vi "实时小时数据单参数上传.vi"(11 "错误输入（无错误）":errorcluster) -> (4 "数据发送起始时间":timestamp format="%<%.3X\n%Y/%m/%d>T", 15 "error out":errorcluster)   [LabVIEW 2016, in "数据传输系统-03.lvlib"]
uses:
  <vilib>/Utility/config.llb/Read Key (String).vi
  <vilib>/Utility/config.llb/Write Key (String).vi
  <vilib>/Utility/config.llb/NI_LVConfig.lvlib
panel:
  out "数据拆分":bool
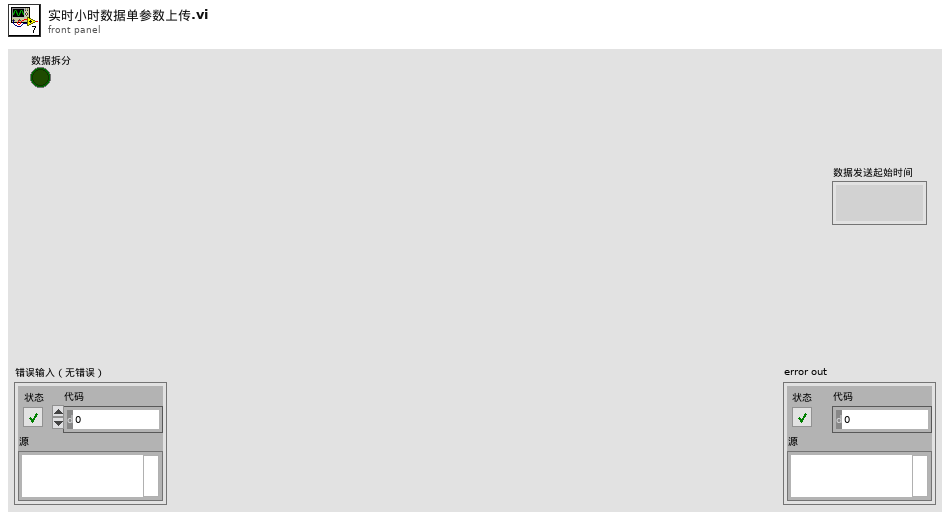
[diagram p1: front panel]
types:
  T1 = cluster{"CODMn":string, "CODCr":string, "DO":string, "铜":string, "PH":string, "氨氮":string, "比电导率":string, "水温":string, "COD":string, "浊度":string, "总氮":string, "总磷":string, "叶绿素a":string, "藻密度":string, "水位":string, "流速":string, "瞬时流量":string, "累积流量":string, "亚硝酸盐":string, "硫化物":string, "ORP":string, "铅":string, "镉":string, "锌":string, "镍":string, "锰":string, "汞":string, "气温":string, "气压":string, "风速":string, "风向":string, "盐度":string, "磷酸盐":string, "硝氮":string, "氟化物":string}
  T2 = cluster{"setini":string, "sysini":string, "hechaini":string, "actualwrite":string, "actualread":string, "datasent":string, "反控命令信息队列":string, "反控与仪器交互":string}
  T3 = typedef "NI_LVConfig.lvlib/Config Data RefNum.ctl" = refnum<k1>
  T4 = cluster{"time1":string, "time2":string, "time3":string, "time4":string, "time5":string, "time6":string, "time7":string, "time8":string, "time9":string, "time10":string, "time11":string, "time12":string, "time13":string, "time14":string, "time15":string, "time16":string, "time17":string, "time18":string, "time19":string, "time20":string, "time21":string, "time22":string, "time23":string, "time24":string, "time25":string, "time26":string, "time27":string, "time28":string, "time29":string, "time30":string, "time31":string, "time32":string, "time33":string, "time34":string, "time35":string}
  T5 = cluster{"水样数据索引[0]":string, "水样数据索引[1]":string, "水样数据索引[2]":string, "水样数据索引[3]":string, "水样数据索引[4]":string, "水样数据索引[5]":string, "水样数据索引[6]":string, "水样数据索引[7]":string, "水样数据索引[8]":string, "水样数据索引[9]":string, "水样数据索引[10]":string, "水样数据索引[11]":string, "水样数据索引[12]":string, "水样数据索引[13]":string, "水样数据索引[14]":string, "水样数据索引[15]":string, "水样数据索引[16]":string, "水样数据索引[17]":string, "水样数据索引[18]":string, "水样数据索引[19]":string, "水样数据索引[20]":string, "水样数据索引[21]":string, "水样数据索引[22]":string, "水样数据索引[23]":string, "水样数据索引[24]":string, "水样数据索引[25]":string, "水样数据索引[26]":string, "水样数据索引[27]":string, "水样数据索引[28]":string, "水样数据索引[29]":string, "水样数据索引[30]":string, "水样数据索引[31]":string, "水样数据索引[32]":string, "水样数据索引[33]":string, "水样数据索引[34]":string}
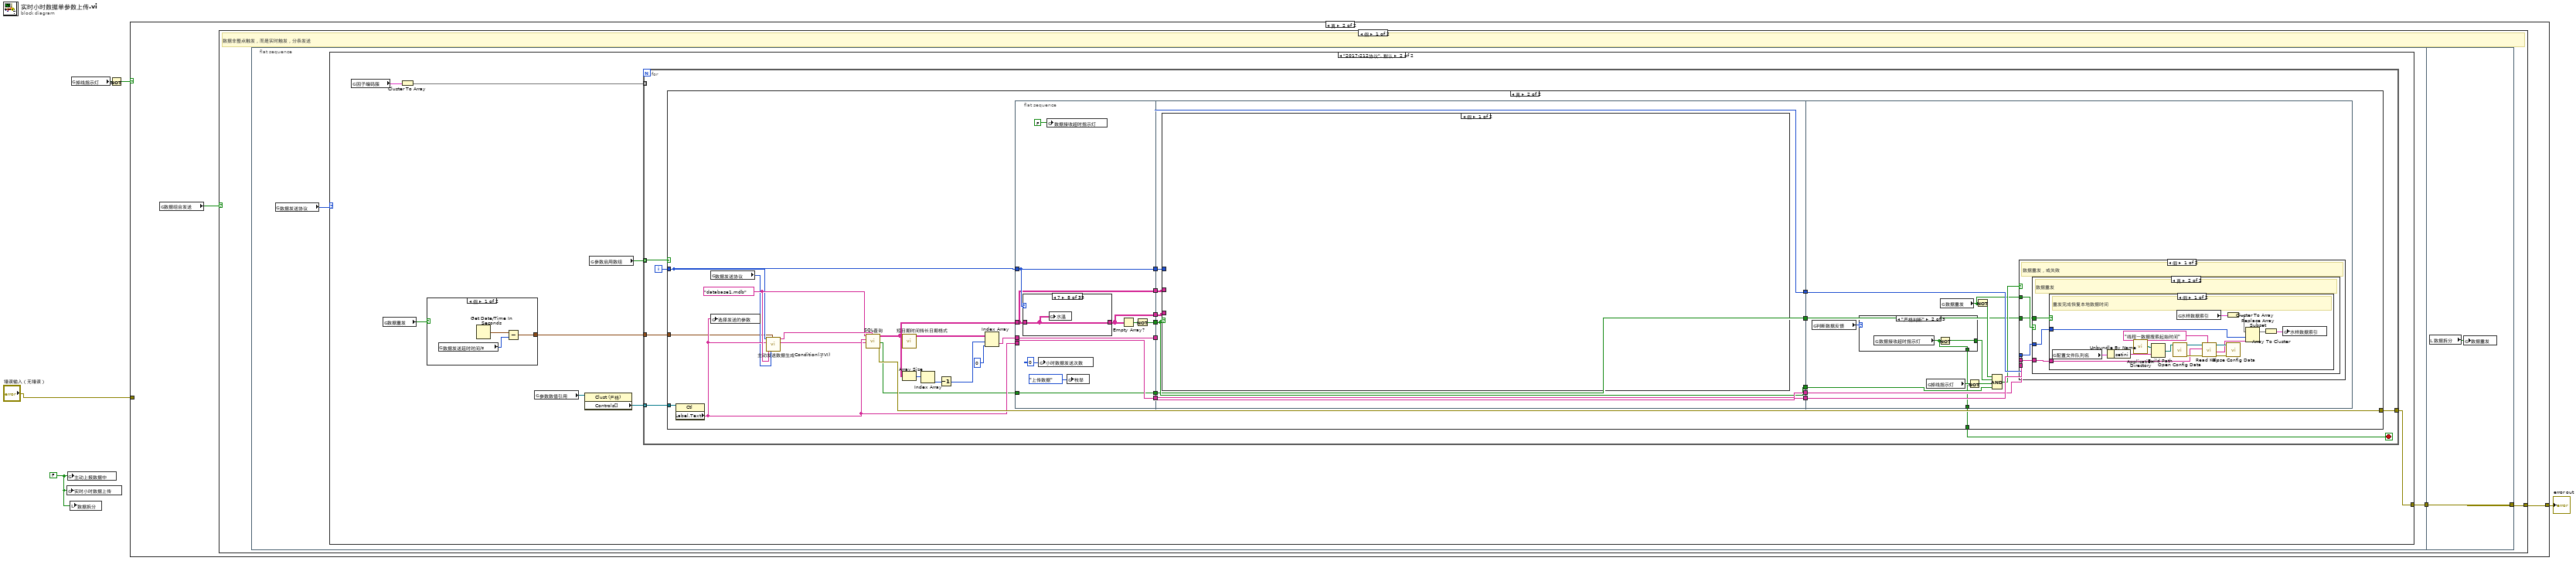
[diagram p0: block diagram]
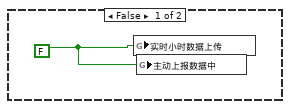
[diagram p2: hidden frame]
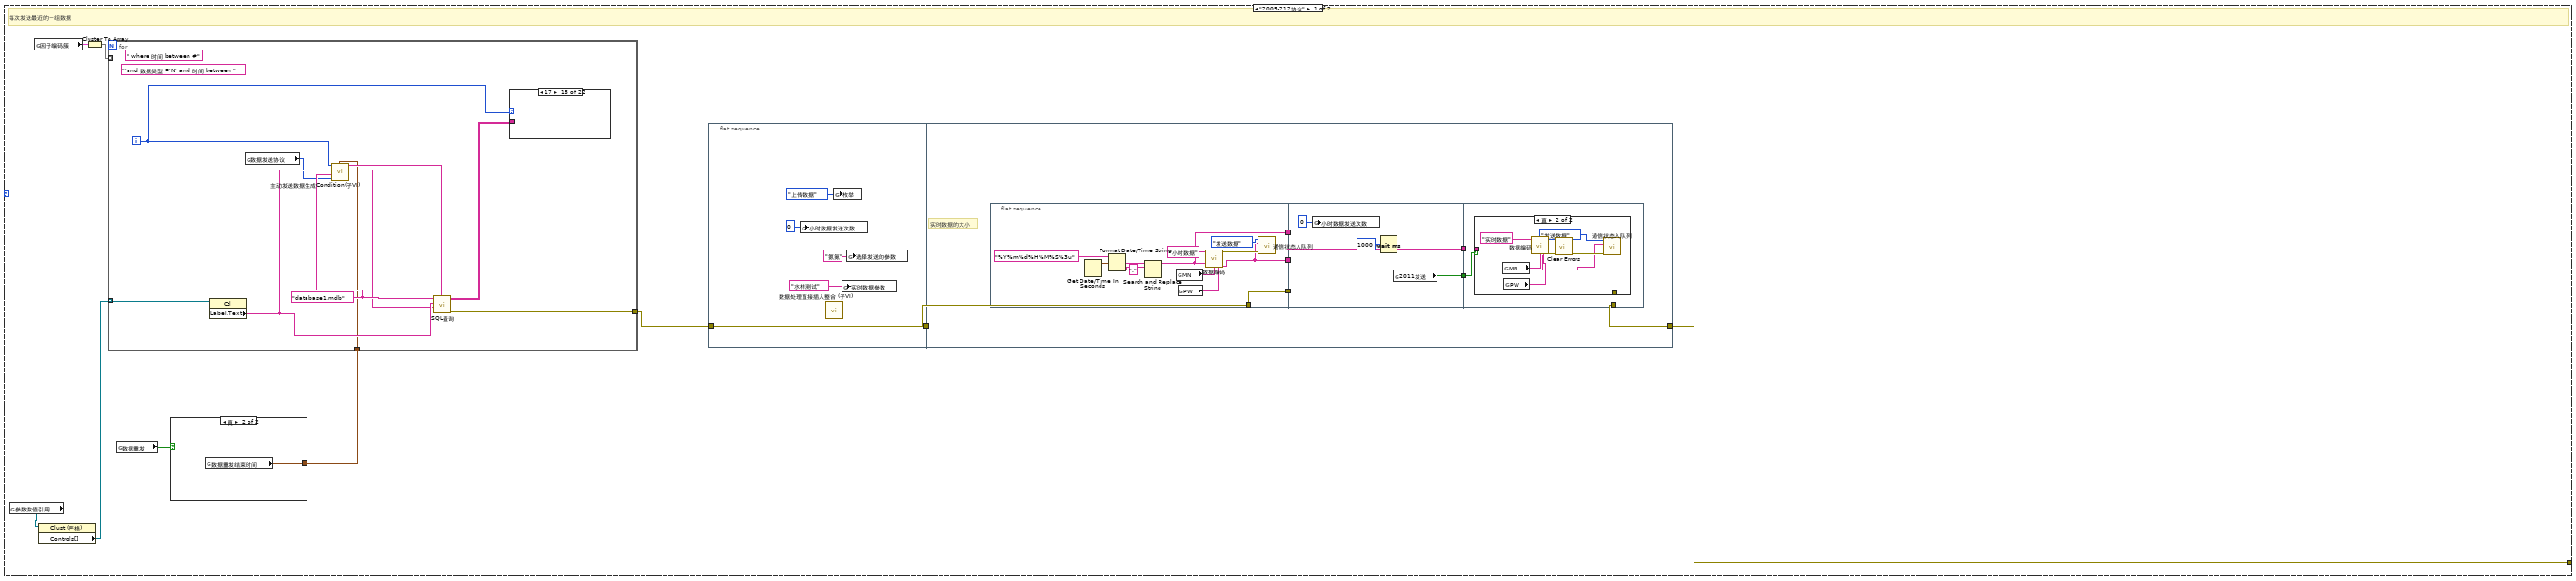
[diagram p3: hidden frame]
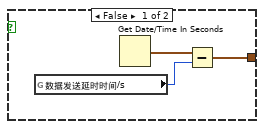
[diagram p4: hidden frame]
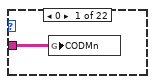
[diagram p6: hidden frame]
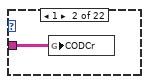
[diagram p7: hidden frame]
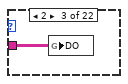
[diagram p8: hidden frame]
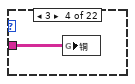
[diagram p9: hidden frame]
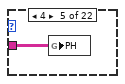
[diagram p10: hidden frame]
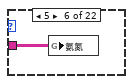
[diagram p11: hidden frame]
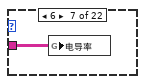
[diagram p12: hidden frame]
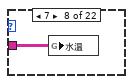
[diagram p13: hidden frame]
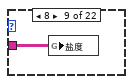
[diagram p14: hidden frame]
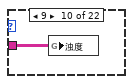
[diagram p15: hidden frame]
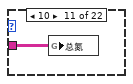
[diagram p16: hidden frame]
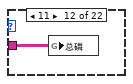
[diagram p17: hidden frame]
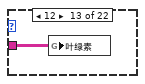
[diagram p18: hidden frame]
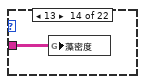
[diagram p19: hidden frame]
diagram:
  w1 = FALSE ("小时数据上传")
  n1 = global write "全局1.vi" "实时小时数据上传"(w1) -> ()
  n2 = global write "全局 数据发送重叠.vi" "主动上报数据中"(w1) -> ()
  n3 = local write "数据拆分"(w1) -> ()
  n4 = global read "全局 数据发送重叠.vi" "掉线指示灯"() -> (w5:bool)
  n5 = Not(x=w5) -> (.not. x?=w4:bool)
  n6 = case shown="真" w4 {
    tunnel: [_ w8] -> w3
    tunnel: "错误输入（无错误）" -> [_ _]
    frame False {
      w6 = FALSE ("小时数据上传")
      n7 = global write "全局1.vi" "实时小时数据上传"(w6) -> ()
      n8 = global write "全局 数据发送重叠.vi" "主动上报数据中"(w6) -> ()
    }
    frame True {
      n9 = global read "断电保存全局.vi" "数据组合发送"() -> (w7:bool)
      n10 = case shown="假" w7 {
        tunnel: [w9 _] -> w8
        frame False {
          # "数据非整点触发，而是实时触发，分条发送"
          n11 = flat-sequence {
            tunnel: [w12] -> w10
            tunnel: [w353] -> w9
            tunnel: w10 -> [w353]
            frame #0 {
              n12 = global read "断电保存全局.vi" "数据发送协议"() -> (w11:enum16{"2005-212协议", "2017-212协议"})
              n13 = case shown="\"2017-212协议\", 默认" w11 {
                tunnel: [w17 w99] -> w12
                frame "2005-212协议" {
                  # "每次发送最近的一组数据"
                  n14 = global read "断电保存全局.vi" "参数数值引用"() -> (w15:refnum<vi>)
                  n15 = global read "断电保存全局.vi" "因子编码簇"() -> (w16:T1)
                  n16 = property class="Clust (严格)"(reference=w15) -> ("Controls[]"=w18:refnum<vi>[])  [unwired: 1 in, 2 out]
                  n17 = Cluster To Array(cluster=w16) -> (array=w21:string[])
                  n18 = global read "断电保存全局.vi" "数据重发"() -> (w14:bool)
                  n19 = case shown="真" w14 {
                    tunnel: [w22 w25] -> w13
                    frame False {
                      n20 = global read "断电保存全局.vi" "数据发送延时时间/s"() -> (w23:i32)
                      n21 = Get Date/Time In Seconds() -> (seconds since 1Jan1904=w24:timestamp)
                      n22 = Subtract(x=w24, y=w23) -> (x-y=w22:timestamp)
                    }
                    frame True {
                      n23 = global read "断电保存全局.vi" "数据重发结束时间"() -> (w25:timestamp)
                    }
                  }
                  n24 = for {
                    tunnel: w21 -> [_] mode=indexing
                    tunnel: [w75] -> w20
                    tunnel: w18 -> [w70] mode=indexing
                    tunnel: w13 -> [w67]
                    i -> [w68]
                    (unwired) " where 时间 between #"
                    w73 = "database1.mdb" ("database")
                    (unwired) "'and 数据类型 ='N' and 时间 between "
                    n25 = property class="Ctl"(reference=w70) -> ("Label.Text"=w74:string)  [unwired: 1 in, 2 out]
                    n26 = global read "断电保存全局.vi" "数据发送协议"() -> (w71:enum16{"2005-212协议", "2017-212协议"})
                    n27 = call "主动发送数据生成Condition(子VI).vi"("结束时间"=w67, "数据发送协议"=w71, "database"=w73, "Label.Text"=w74, "数值"=w68) -> ("columns"=w66:string[], "CONDITION"=w72:string)  [unwired: 5 in]
                    n28 = call "SQL查询.vi"("condition"=w72, "columns"=w66, "table输入"=w74, "database"=w73) -> ("error out"=w75:errorcluster, "data"=w69:string[][])  [unwired: 4 in, 2 out]
                    n29 = case shown="17" w68 {
                      tunnel: w69 -> [w76 w77 w78 w79 w80 w81 w82 w83 w84 w85 w86 w87 w88 w89 _ _ _ _ w90 w91 w92 _]
                      frame 0 {
                        n30 = global write "全局 所有参数.vi" "CODMn"(w76) -> ()
                      }
                      frame 1 {
                        n31 = global write "全局 所有参数.vi" "CODCr"(w77) -> ()
                      }
                      frame 2 {
                        n32 = global write "全局 所有参数.vi" "DO"(w78) -> ()
                      }
                      frame 3 {
                        n33 = global write "全局 所有参数.vi" "铜"(w79) -> ()
                      }
                      frame 4 {
                        n34 = global write "全局 所有参数.vi" "PH"(w80) -> ()
                      }
                      frame 5 {
                        n35 = global write "全局 所有参数.vi" "氨氮"(w81) -> ()
                      }
                      frame 6 {
                        n36 = global write "全局 所有参数.vi" "电导率"(w82) -> ()
                      }
                      frame 7 {
                        n37 = global write "全局 所有参数.vi" "水温"(w83) -> ()
                      }
                      frame 8 {
                        n38 = global write "全局 所有参数.vi" "盐度"(w84) -> ()
                      }
                      frame 9 {
                        n39 = global write "全局 所有参数.vi" "浊度"(w85) -> ()
                      }
                      frame 10 {
                        n40 = global write "全局 所有参数.vi" "总氮"(w86) -> ()
                      }
                      frame 11 {
                        n41 = global write "全局 所有参数.vi" "总磷"(w87) -> ()
                      }
                      frame 12 {
                        n42 = global write "全局 所有参数.vi" "叶绿素"(w88) -> ()
                      }
                      frame 13 {
                        n43 = global write "全局 所有参数.vi" "藻密度"(w89) -> ()
                      }
                      frame 14 {
                      }
                      frame 15 {
                      }
                      frame 16 {
                      }
                      frame 17 {
                      }
                      frame 18 {
                        n44 = global write "全局 所有参数.vi" "亚硝酸盐"(w90) -> ()
                      }
                      frame 19 {
                        n45 = global write "全局 所有参数.vi" "硫化物"(w91) -> ()
                      }
                      frame 20 {
                        n46 = global write "全局 所有参数.vi" "ORP"(w92) -> ()
                      }
                      frame 21, Default {
                      }
                    }
                  }
                  n47 = flat-sequence {
                    tunnel: w20 -> [w26]
                    tunnel: [w26] -> w19
                    tunnel: w19 -> [w35]
                    tunnel: [w34] -> w17
                    frame #0 {
                      n48 = global write "全局 小时数据发送次数.vi" "小时数据发送次数"(0 ("小时数据发送次数")) -> ()
                      n49 = call "数据处理直接插入整合 (子VI).vi"() -> ()  [unwired: 12 in]
                      n50 = global write "全局1.vi" "枚举"(enum16{"返回请求应答", "上传数据", "返回执行结果"}."上传数据" ("枚举")) -> ()
                      n51 = global write "全局 实时数据参数.vi" "实时数据参数"("水样测试" ("实时数据参数")) -> ()
                      n52 = global write "全局 水样时间.vi" "选择发送的参数"("氨氮" ("选择发送的参数")) -> ()
                    }
                    frame #1 {
                      # "实时数据的大小"
                      n53 = flat-sequence {
                        tunnel: [w38] -> w37
                        tunnel: [w41] -> w36
                        tunnel: w35 -> [w41]
                        tunnel: [w40] -> w33
                        tunnel: w37 -> [_]
                        tunnel: w36 -> [_]
                        tunnel: w33 -> [w51]
                        tunnel: [w51] -> w32
                        tunnel: [w50] -> w31
                        tunnel: [w56] -> w34
                        tunnel: w32 -> [w55]
                        tunnel: w31 -> [w54]
                        frame #0 {
                          n54 = Get Date/Time In Seconds() -> (seconds since 1Jan1904=w47:timestamp)
                          n55 = Format Date/Time String(time format string (%c)="%Y%m%d%H%M%S%3u" ("时间格式字符串(%c)"), seconds (now)=w47) -> (date/time string=w48:string)  [unwired: 1 in]
                          n56 = Search and Replace String(input string=w48, search string="." ("搜索字符串")) -> (result string=w40:string)  [unwired: 6 in, 3 out]
                          n57 = global read "断电保存全局.vi" "MN"() -> (w44:string)
                          n58 = global read "断电保存全局.vi" "PW"() -> (w43:string)
                          n59 = call "数据编码.vi"("table输入"="小时数据" ("新元素/子数组"), "QN"=w40, "MN"=w44, "PW"=w43) -> ("错误常量"=w42:errorcluster, "通讯包字符串"=w38:string)  [unwired: 10 in]
                          n60 = call "通信状态入队列.vi"("错误输入（无错误）"=w42, "发送报文"=w38, "枚举"=enum16{"打开连接", "发送数据", "读取数据", "数据处理", "关闭连接"}."发送数据") -> ()  [unwired: 8 in, 1 out]
                        }
                        frame #1 {
                          n61 = global write "全局 小时数据发送次数.vi" "小时数据发送次数"(0 ("小时数据发送次数")) -> ()
                          n62 = Wait (ms)(milliseconds to wait=u32 1000 ("等待时间（毫秒）")) -> ()  [unwired: 1 out]
                          n63 = global read "断电保存全局.vi" "2011发送"() -> (w50:bool)
                        }
                        frame #2 {
                          n64 = case shown="真" w54 {
                            tunnel: [_ w61] -> w56
                            tunnel: w55 -> [_ w60]
                            frame False {
                            }
                            frame True {
                              n65 = global read "断电保存全局.vi" "MN"() -> (w63:string)
                              n66 = global read "断电保存全局.vi" "PW"() -> (w64:string)
                              n67 = call "数据编码.vi"("table输入"="实时数据" ("新元素/子数组"), "QN"=w60, "MN"=w63, "PW"=w64) -> ("错误常量"=w62:errorcluster, "通讯包字符串"=w57:string)  [unwired: 10 in]
                              n68 = call <vilib>:"Clear Errors.vi"("error in (no error)"=w62) -> ("error out"=w59:errorcluster)  [unwired: 5 in, 1 out]
                              n69 = call "通信状态入队列.vi"("错误输入（无错误）"=w59, "发送报文"=w57, "枚举"=enum16{"打开连接", "发送数据", "读取数据", "数据处理", "关闭连接"}."发送数据") -> ("错误输出"=w61:errorcluster)  [unwired: 8 in]
                            }
                          }
                        }
                      }
                    }
                  }
                }
                frame "2017-212协议", Default {
                  n70 = global read "断电保存全局.vi" "因子编码簇"() -> (w97:T1)
                  n71 = global read "断电保存全局.vi" "数据重发"() -> (w94:bool)
                  n72 = Cluster To Array(cluster=w97) -> (array=w100:string[])
                  n73 = case shown="假" w94 {
                    tunnel: [w101 w104] -> w93
                    frame False {
                      n74 = global read "断电保存全局.vi" "数据发送延时时间/s"() -> (w102:i32)
                      n75 = Get Date/Time In Seconds() -> (seconds since 1Jan1904=w103:timestamp)
                      n76 = Subtract(x=w103, y=w102) -> (x-y=w101:timestamp)
                    }
                    frame True {
                      n77 = global read "断电保存全局.vi" "数据重发结束时间"() -> (w104:timestamp)
                    }
                  }
                  n78 = global read "断电保存全局.vi" "参数数值引用"() -> (w96:refnum<vi>)
                  n79 = property class="Clust (严格)"(reference=w96) -> ("Controls[]"=w98:refnum<vi>[])  [unwired: 1 in, 2 out]
                  n80 = global read "断电保存全局.vi" "参数启用数组"() -> (w95:bool[])
                  n81 = for {
                    tunnel: w100 -> [_] mode=indexing
                    tunnel: [w110] -> w99
                    tunnel: w98 -> [w108] mode=indexing
                    tunnel: w95 -> [w107] mode=indexing
                    tunnel: w93 -> [w106]
                    i -> [w109]
                    stop <- w105 stop-if-true
                    n82 = case shown="真" w107 {
                      tunnel: [_ w129] -> w110
                      tunnel: w109 -> [_ w120]
                      tunnel: w108 -> [_ w119]
                      tunnel: w106 -> [_ w116]
                      tunnel: [_ w114] -> w105
                      frame False {
                      }
                      frame True {
                        w128 = "database1.mdb" ("database")
                        n83 = property class="Ctl"(reference=w119) -> ("Label.Text"=w127:string)  [unwired: 1 in, 2 out]
                        n84 = global read "断电保存全局.vi" "数据发送协议"() -> (w126:enum16{"2005-212协议", "2017-212协议"})
                        n85 = global write "全局 水样时间.vi" "选择发送的参数"(w127) -> ()
                        n86 = call "主动发送数据生成Condition(子VI).vi"("结束时间"=w116, "数据发送协议"=w126, "database"=w128, "Label.Text"=w127, "数值"=w120) -> ("columns"=w118:string[], "CONDITION"=w132:string)  [unwired: 5 in]
                        n87 = call "SQL查询.vi"("condition"=w132, "columns"=w118, "table输入"=w127, "database"=w128) -> ("error out"=w129:errorcluster, "拆分数据"=w112:bool, "data"=w123:string[][])  [unwired: 4 in, 1 out]
                        n88 = call "短日期时间转长日期格式.vi"("data"=w123) -> ("输出数组"=w131:string[][])  [unwired: 10 in]
                        n89 = Array Size(array=w123) -> (size(s)=w125:i32[])
                        n90 = Index Array(array=w125) -> (element=w124:i32)  [unwired: 1 in]
                        n91 = Decrement(x=w124) -> (x-1=w122:i32)
                        n92 = Index Array(array=w131, index (row)=w122, index (col)=0 ("禁用的索引 (列)")) -> (element=w130:string)
                        n93 = flat-sequence {
                          tunnel: [w144] -> w140
                          tunnel: [w143] -> w139
                          tunnel: w123 -> [w142]
                          tunnel: w120 -> [w147]
                          tunnel: w127 -> [w149]
                          tunnel: [w149] -> w138
                          tunnel: w130 -> [w148]
                          tunnel: [w148] -> w137
                          tunnel: [w147] -> w136
                          tunnel: [w142] -> w115
                          tunnel: [w141] -> w113
                          tunnel: w112 -> [w141]
                          tunnel: w140 -> [w189]
                          tunnel: w139 -> [w193]
                          tunnel: [w192] -> w135
                          tunnel: w138 -> [w192]
                          tunnel: [w191] -> w134
                          tunnel: w137 -> [w191]
                          tunnel: [w190] -> w133
                          tunnel: w136 -> [w190]
                          tunnel: [w189] -> w117
                          tunnel: w115 -> [w188]
                          tunnel: w113 -> [w187]
                          tunnel: [w187] -> w111
                          tunnel: w135 -> [w302]
                          tunnel: w134 -> [w301]
                          tunnel: w133 -> [w300]
                          tunnel: w117 -> [w299]
                          tunnel: [w291] -> w114
                          tunnel: w111 -> [w290]
                          frame #0 {
                            n94 = case shown="7" w147 {
                              tunnel: w142 -> [w152 w153 w154 w155 w156 w157 w158 w159 w160 w161 w162 w163 w164 w165 _ _ _ _ w170 w171 w172 w173 w174 w175 w176 w177 w178 _ _ _ _ w183 w184 w185 w186]
                              tunnel: [w152 w153 w154 w155 w156 w157 w158 w159 w160 w161 w162 w163 w164 w165 w166 w167 w168 w169 w170 w171 w172 w173 w174 w175 w176 w177 w178 w179 w180 w181 w182 w183 w184 w185 w186] -> w143
                              frame 0, Default {
                                n95 = global write "全局 所有参数.vi" "CODMn"(w152) -> ()
                              }
                              frame 1 {
                                n96 = global write "全局 所有参数.vi" "CODCr"(w153) -> ()
                              }
                              frame 2 {
                                n97 = global write "全局 所有参数.vi" "DO"(w154) -> ()
                              }
                              frame 3 {
                                n98 = global write "全局 所有参数.vi" "铜"(w155) -> ()
                              }
                              frame 4 {
                                n99 = global write "全局 所有参数.vi" "PH"(w156) -> ()
                              }
                              frame 5 {
                                n100 = global write "全局 所有参数.vi" "氨氮"(w157) -> ()
                              }
                              frame 6 {
                                n101 = global write "全局 所有参数.vi" "电导率"(w158) -> ()
                              }
                              frame 7 {
                                n102 = global write "全局 所有参数.vi" "水温"(w159) -> ()
                              }
                              frame 8 {
                                n103 = global write "全局 所有参数.vi" "盐度"(w160) -> ()
                              }
                              frame 9 {
                                n104 = global write "全局 所有参数.vi" "浊度"(w161) -> ()
                              }
                              frame 10 {
                                n105 = global write "全局 所有参数.vi" "总氮"(w162) -> ()
                              }
                              frame 11 {
                                n106 = global write "全局 所有参数.vi" "总磷"(w163) -> ()
                              }
                              frame 12 {
                                n107 = global write "全局 所有参数.vi" "叶绿素"(w164) -> ()
                              }
                              frame 13 {
                                n108 = global write "全局 所有参数.vi" "藻密度"(w165) -> ()
                              }
                              frame 14 {
                                n109 = global read "全局 所有参数.vi" "水位"() -> (w166:string[][])
                              }
                              frame 15 {
                                n110 = global read "全局 所有参数.vi" "流速"() -> (w167:string[][])
                              }
                              frame 16 {
                                n111 = global read "全局 所有参数.vi" "瞬时流量"() -> (w168:string[][])
                              }
                              frame 17 {
                                n112 = global read "全局 所有参数.vi" "累积流量"() -> (w169:string[][])
                              }
                              frame 18 {
                                n113 = global write "全局 所有参数.vi" "亚硝酸盐"(w170) -> ()
                              }
                              frame 19 {
                                n114 = global write "全局 所有参数.vi" "硫化物"(w171) -> ()
                              }
                              frame 20 {
                                n115 = global write "全局 所有参数.vi" "ORP"(w172) -> ()
                              }
                              frame 21 {
                                n116 = global write "全局 所有参数.vi" "铅"(w173) -> ()
                              }
                              frame 22 {
                                n117 = global write "全局 所有参数.vi" "镉"(w174) -> ()
                              }
                              frame 23 {
                                n118 = global write "全局 所有参数.vi" "锌"(w175) -> ()
                              }
                              frame 24 {
                                n119 = global write "全局 所有参数.vi" "镍"(w176) -> ()
                              }
                              frame 25 {
                                n120 = global write "全局 所有参数.vi" "锰"(w177) -> ()
                              }
                              frame 26 {
                                n121 = global write "全局 所有参数.vi" "汞"(w178) -> ()
                              }
                              frame 27 {
                                n122 = global read "全局 所有参数.vi" "气温"() -> (w179:string[][])
                              }
                              frame 28 {
                                n123 = global read "全局 所有参数.vi" "气压"() -> (w180:string[][])
                              }
                              frame 29 {
                                n124 = global read "全局 所有参数.vi" "风速"() -> (w181:string[][])
                              }
                              frame 30 {
                                n125 = global read "全局 所有参数.vi" "风向"() -> (w182:string[][])
                              }
                              frame 31 {
                                n126 = global write "全局 所有参数.vi" "盐度 2"(w183) -> ()
                              }
                              frame 32 {
                                n127 = global write "全局 所有参数.vi" "磷酸盐"(w184) -> ()
                              }
                              frame 33 {
                                n128 = global write "全局 所有参数.vi" "硝氮"(w185) -> ()
                              }
                              frame 34 {
                                n129 = global write "全局 所有参数.vi" "氟化物"(w186) -> ()
                              }
                            }
                            n130 = global write "全局 小时数据发送次数.vi" "小时数据发送次数"(0 ("小时数据发送次数")) -> ()
                            n131 = global write "全局 数据发送重叠.vi" "数据接收超时指示灯"(FALSE ("数据接收超时指示灯")) -> ()
                            n132 = global write "全局1.vi" "枚举"(enum16{"返回请求应答", "上传数据", "返回执行结果"}."上传数据" ("枚举")) -> ()
                            n133 = Empty Array?(array=w143) -> (empty?=w145:bool)
                            n134 = Not(x=w145) -> (.not. x?=w144:bool)
                          }
                          frame #1 {
                            n135 = case shown="假" w189 {
                              tunnel: w193 -> [_ w198]
                              tunnel: w190 -> [_ w197]
                              tunnel: w188 -> [_ w195]
                              frame False {
                              }
                              frame True {
                                n136 = flat-sequence {
                                tunnel: w198 -> [w201]
                                tunnel: [w201] -> w196
                                tunnel: w195 -> [w199]
                                tunnel: [w199] -> w194
                                tunnel: w197 -> [w203]
                                tunnel: w196 -> [w204]
                                tunnel: w194 -> [w202]
                                frame #0 {
                                w200 = TRUE ("小时数据上传")
                                n137 = global write "全局 数据发送重叠.vi" "主动上报数据中"(w200) -> ()
                                n138 = global write "全局1.vi" "实时小时数据上传"(w200) -> ()
                                }
                                frame #1 {
                                n139 = case shown="0, 默认" w203 {
                                selector: w203 -> [w205 _]
                                tunnel: w203 -> [_ w236]
                                tunnel: w204 -> [w208 w235]
                                tunnel: w202 -> [w207 w234]
                                frame 14..17, 27..30 {
                                n140 = for {
                                tunnel: [w232] -> w209
                                tunnel: w205 -> [w231]
                                tunnel: w208 -> [_] mode=indexing
                                i -> [w233]
                                stop <- w230 stop-if-true
                                n141 = call "小时数据发送 (子VI).vi"("数值"=w231) -> ("error out"=w232:errorcluster, "超时退出"=w230:bool)  [unwired: 9 in]
                                n142 = global write "全局 小时数据发送次数.vi" "小时数据发送次数"(w233) -> ()
                                }
                                n143 = global read "断电保存全局.vi" "2011发送"() -> (w206:bool)
                                n144 = case shown="真" w206 {
                                tunnel: w209 -> [_ w214]
                                tunnel: w205 -> [_ w213]
                                tunnel: w207 -> [_ w212]
                                tunnel: w205 -> [_ w210]
                                frame False {
                                }
                                frame True {
                                n145 = flat-sequence {
                                tunnel: w214 -> [w218]
                                tunnel: [w218] -> w215
                                tunnel: w213 -> [w217]
                                tunnel: w212 -> [w216]
                                tunnel: [w216] -> w211
                                frame #0 {
                                n146 = case shown="27" w217 {
                                tunnel: w216 -> [_ w219 w220 w221 w222 w223 w224 w225 w226]
                                frame 0, Default {
                                }
                                frame 14 {
                                n147 = global write "全局 所有参数.vi" "水位"(w219) -> ()
                                }
                                frame 15 {
                                n148 = global write "全局 所有参数.vi" "流速"(w220) -> ()
                                }
                                frame 16 {
                                n149 = global write "全局 所有参数.vi" "瞬时流量"(w221) -> ()
                                }
                                frame 17 {
                                n150 = global write "全局 所有参数.vi" "累积流量"(w222) -> ()
                                }
                                frame 27 {
                                n151 = global write "全局 所有参数.vi" "气温"(w223) -> ()
                                }
                                frame 28 {
                                n152 = global write "全局 所有参数.vi" "气压"(w224) -> ()
                                }
                                frame 29 {
                                n153 = global write "全局 所有参数.vi" "风速"(w225) -> ()
                                }
                                frame 30 {
                                n154 = global write "全局 所有参数.vi" "风向"(w226) -> ()
                                }
                                }
                                }
                                }
                                n155 = for {
                                tunnel: w215 -> [_]
                                tunnel: w211 -> [_] mode=indexing
                                tunnel: w210 -> [w228]
                                i -> [w229]
                                stop <- w227 stop-if-true
                                n156 = global write "全局 小时数据发送次数.vi" "小时数据发送次数"(w229) -> ()
                                n157 = call "实时数据发送 (子VI).vi"("数值"=w228) -> ("超时退出"=w227:bool)  [unwired: 10 in]
                                }
                                }
                                }
                                }
                                frame 0, Default {
                                n158 = for {
                                tunnel: w236 -> [w239]
                                tunnel: w235 -> [w245] mode=indexing
                                tunnel: w234 -> [w241]
                                i -> [w240]
                                stop <- w237 stop-if-true
                                n159 = Index Array(array=w245, index #1=1 ("索引"), index #2=2 ("索引")) -> (element #1=w238:string, element #2=w242:string)
                                n160 = global write "全局 小时数据发送次数.vi" "小时数据发送次数"(w240) -> ()
                                n161 = case shown="\"水样测试\"" w238 {
                                tunnel: w239 -> [_ w249 _ _ _]
                                tunnel: w242 -> [_ w248 w281 w284 w287]
                                tunnel: w241 -> [_ w247 _ _ _]
                                tunnel: [_ w246 w280 w283 w286] -> w237
                                frame "假", Default {
                                }
                                frame "水样测试" {
                                n162 = case shown="\"hd\", \"N\", 默认" w248 {
                                tunnel: w249 -> [w253 w274]
                                tunnel: w247 -> [w252 w273]
                                tunnel: [w250 w271] -> w246
                                frame "M" {
                                n163 = global read "断电保存全局.vi" "2011发送"() -> (w251:bool)
                                n164 = case shown="真" w251 {
                                tunnel: w253 -> [_ w256]
                                tunnel: w252 -> [_ w255]
                                tunnel: [_ w254] -> w250
                                frame False {
                                }
                                frame True {
                                n165 = flat-sequence {
                                tunnel: w256 -> [w258]
                                tunnel: w255 -> [w259]
                                tunnel: [w258] -> w257
                                tunnel: w257 -> [w269]
                                tunnel: [w268] -> w254
                                frame #0 {
                                n166 = case shown="14" w258 {
                                tunnel: w259 -> [_ w260 w261 w262 w263 w264 w265 w266 w267]
                                frame 0, Default {
                                }
                                frame 14 {
                                n167 = global write "全局 所有参数.vi" "水位"(w260) -> ()
                                }
                                frame 15 {
                                n168 = global write "全局 所有参数.vi" "流速"(w261) -> ()
                                }
                                frame 16 {
                                n169 = global write "全局 所有参数.vi" "瞬时流量"(w262) -> ()
                                }
                                frame 17 {
                                n170 = global write "全局 所有参数.vi" "累积流量"(w263) -> ()
                                }
                                frame 27 {
                                n171 = global write "全局 所有参数.vi" "气温"(w264) -> ()
                                }
                                frame 28 {
                                n172 = global write "全局 所有参数.vi" "气压"(w265) -> ()
                                }
                                frame 29 {
                                n173 = global write "全局 所有参数.vi" "风速"(w266) -> ()
                                }
                                frame 30 {
                                n174 = global write "全局 所有参数.vi" "风向"(w267) -> ()
                                }
                                }
                                }
                                frame #1 {
                                n175 = call "实时数据发送 (子VI).vi"("数值"=w269) -> ("超时退出"=w268:bool)  [unwired: 10 in]
                                }
                                }
                                }
                                }
                                }
                                frame "hd", "N", Default {
                                n176 = call "小时数据发送 (子VI).vi"("数值"=w274) -> ("error out"=w272:errorcluster, "超时退出"=w270:bool)  [unwired: 9 in]
                                n177 = global read "断电保存全局.vi" "2011发送"() -> (w275:bool)
                                n178 = case shown="真" w275 {
                                tunnel: w274 -> [_ w279]
                                tunnel: w273 -> [_ _]
                                tunnel: w272 -> [_ _]
                                tunnel: [_ w276] -> w271
                                tunnel: w270 -> [_ w278]
                                frame False {
                                }
                                frame True {
                                n179 = call "实时数据发送 (子VI).vi"("数值"=w279) -> ("超时退出"=w277:bool)  [unwired: 10 in]
                                n180 = Or(x=w278, y=w277) -> (x .or. y?=w276:bool)
                                }
                                }
                                }
                                }
                                }
                                frame "空白测试", "零点核查" {
                                n181 = case shown="\"N\", 默认" w281 {
                                tunnel: [_ w282] -> w280
                                frame "M" {
                                }
                                frame "N", Default {
                                n182 = call "零点核查数据发送 (子VI).vi"() -> ("超时退出"=w282:bool)  [unwired: 11 in]
                                }
                                }
                                }
                                frame "跨度核查" {
                                n183 = case shown="\"N\", 默认" w284 {
                                tunnel: [_ w285] -> w283
                                frame "M" {
                                }
                                frame "N", Default {
                                n184 = call "跨度核查数据发送 (子VI).vi"() -> ("超时退出"=w285:bool)  [unwired: 11 in]
                                }
                                }
                                }
                                frame "标样核查" {
                                n185 = case shown="\"N\", 默认" w287 {
                                tunnel: [_ w288] -> w286
                                frame "M" {
                                }
                                frame "N", Default {
                                n186 = call "标样核查数据发送(子VI).vi"() -> ("超时退出"=w288:bool)  [unwired: 11 in]
                                }
                                }
                                }
                                }
                                }
                                }
                                }
                                }
                                frame #2 {
                                w289 = FALSE ("小时数据上传")
                                n187 = global write "全局 数据发送重叠.vi" "主动上报数据中"(w289) -> ()
                                n188 = global write "全局1.vi" "实时小时数据上传"(w289) -> ()
                                }
                                }
                              }
                            }
                          }
                          frame #2 {
                            n189 = global read "断电保存全局.vi" "判断数据反馈"() -> (w296:enum16{"非严格判断", "严格判断", "不判断"})
                            n190 = case shown="\"严格判断\"" w296 {
                              tunnel: [TRUE w306 TRUE] -> w295
                              tunnel: [FALSE ("数据接收超时指示灯") w305 FALSE ("数据接收超时指示灯")] -> w291
                              frame "非严格判断", Default {
                              }
                              frame "严格判断" {
                                n191 = global read "全局 数据发送重叠.vi" "数据接收超时指示灯"() -> (w305:bool)
                                n192 = Not(x=w305) -> (.not. x?=w306:bool)
                              }
                              frame "不判断" {
                              }
                            }
                            n193 = global read "全局 数据发送重叠.vi" "掉线指示灯"() -> (w298:bool)
                            n194 = global read "断电保存全局.vi" "数据重发"() -> (w292:bool)
                            n195 = Not(x=w298) -> (.not. x?=w297:bool)
                            n196 = Not(x=w292) -> (.not. x?=w293:bool)
                            n197 = Compound Arithmetic op=AND ("复合运算")(w293, w295, w297, w299) -> (w294:bool)
                            n198 = case shown="假" w294 {
                              tunnel: w301 -> [_ w343]
                              tunnel: w300 -> [w310 w337]
                              tunnel: w302 -> [w312 w344]
                              tunnel: w292 -> [w311 _]
                              tunnel: w290 -> [w309 _]
                              frame False {
                                # "数据重发，或失败"
                                n199 = case shown="真" w311 {
                                tunnel: w312 -> [_ w315]
                                tunnel: w310 -> [_ w314]
                                tunnel: w309 -> [_ w313]
                                frame False {
                                # "数据发送失败"
                                }
                                frame True {
                                # "数据重发"
                                n200 = case shown="假" w313 {
                                tunnel: w315 -> [w318 _]
                                tunnel: w314 -> [w316 _]
                                frame False {
                                # "重发完成恢复本地数据时间"
                                n201 = global read "断电保存全局.vi" "配置文件队列名"() -> (w325:T2)
                                n202 = Unbundle By Name(w325) -> ("setini"=w326:string)
                                n203 = call <vilib>:"Application Directory.vi"() -> ("Application Directory"=w319:path)
                                n204 = Build Path(base path=w319, name or relative path=w326) -> (appended path=w320:path)
                                n205 = call <vilib>:"Open Config Data.vi"("configuration file path"=w320) -> ("error out"=w327:errorcluster, "refnum"=w321:T3)  [unwired: 8 in, 1 out]
                                n206 = global read "全局 水样时间.vi" "水样数据索引"() -> (w328:T4)
                                n207 = call-poly <vilib>:"Read Key.vi"("section"="线程一数据搜索起始时间", "error in (no error)"=w327, "key"=w318, "refnum"=w321) -> ("error out"=w324:errorcluster, "value"=w317:string, "refnum out"=w323:T3)  [unwired: 4 in, 1 out]
                                n208 = Cluster To Array(cluster=w328) -> (array=w329:string[])
                                n209 = call <vilib>:"Close Config Data.vi"("error in (no error)"=w324, "refnum"=w323) -> ()  [unwired: 8 in, 2 out]
                                n210 = Replace Array Subset(array=w329, new element=w317, index=w316) -> (w330:string[])
                                n211 = Array To Cluster(array=w330) -> (cluster=w331:T5)
                                n212 = global write "全局 水样时间.vi" "水样数据索引"(w331) -> ()
                                }
                                frame True {
                                # "数据拆分，继续重发"
                                "数据拆分" <- TRUE
                                }
                                }
                                }
                                }
                              }
                              frame True {
                                # "保存本地"
                                n213 = global read "断电保存全局.vi" "配置文件队列名"() -> (w334:T2)
                                n214 = call "日期时间字符串转换分钟数加一.vi"("枚举"=enum16{"分钟数加一", "秒数加一", "小时数加一"}."秒数加一", "data[0]"=w343) -> ("日期/时间字符串"=w336:string)  [unwired: 9 in]
                                n215 = Unbundle By Name(w334) -> ("setini"=w333:string)
                                n216 = global read "全局 水样时间.vi" "水样数据索引"() -> (w338:T4)
                                n217 = call <vilib>:"Application Directory.vi"() -> ("Application Directory"=w345:path)
                                n218 = Build Path(base path=w345, name or relative path=w333) -> (appended path=w346:path)
                                n219 = Cluster To Array(cluster=w338) -> (array=w339:string[])
                                n220 = call <vilib>:"Open Config Data.vi"("configuration file path"=w346) -> ("error out"=w348:errorcluster, "refnum"=w347:T3)  [unwired: 8 in, 1 out]
                                n221 = call "时间日期字符串至时间标识转换.vi"("时间日期字符串"=w336) -> ("时间标识"=→"数据发送起始时间":timestamp)  [unwired: 10 in]
                                n222 = call-poly <vilib>:"Write Key.vi"("section"="线程一数据搜索起始时间", "error in (no error)"=w348, "value"=w336, "key"=w344, "refnum"=w347) -> ("error out"=w350:errorcluster, "refnum out"=w349:T3)  [unwired: 4 in, 1 out]
                                n223 = Replace Array Subset(array=w339, new element=w336, index=w337) -> (w340:string[])
                                n224 = Array To Cluster(array=w340) -> (cluster=w341:T5)
                                n225 = call <vilib>:"Close Config Data.vi"("error in (no error)"=w350, "refnum"=w349) -> ()  [unwired: 8 in, 2 out]
                                n226 = global write "全局 水样时间.vi" "水样数据索引"(w341) -> ()
                              }
                            }
                          }
                        }
                      }
                    }
                  }
                }
              }
            }
            frame #1 {
              n227 = local read "数据拆分"() -> (w352:bool)
              n228 = global write "断电保存全局.vi" "数据重发"(w352) -> ()
            }
          }
        }
        frame True {
          # "数据整点触发，整条发送"
          n229 = flat-sequence {
            frame #0 {
              n230 = global read "断电保存全局.vi" "数据发送通道"() -> (w354:enum16{"TCP", "VISA"})
              n231 = global read "断电保存全局.vi" "MN"() -> (w356:string)
              n232 = global read "断电保存全局.vi" "PW"() -> (w355:string)
              n233 = call "数据全参数一起发送整点触发.vi"("数据发送通道"=w354, "PW"=w355, "MN"=w356) -> ()  [unwired: 8 in]
            }
            frame #1 {
              w357 = FALSE ("主动上报数据中")
              n234 = global write "全局 数据发送重叠.vi" "主动上报数据中"(w357) -> ()
              n235 = global write "全局1.vi" "实时小时数据上传"(w357) -> ()
            }
          }
        }
      }
    }
  }
  "error out" <- w3
